vi "Log Data.vi"(8 "error in (no error)":errorcluster, 9 "variant":variant, 10 "Data REF":T1, 11 "Logging Configuration":T2={"Log File Base Path"=path "", "TDMS File Reference"=refnum, "Reset"=FALSE, "Wait"=0.0, "Start Time"=0.0, "Update Rate"=1, "Channel Names"=[], "System Preset"=variant} {"Update Rate" min=1 max=10 step=1}) -> (0 "error out":errorcluster)   [LabVIEW 2020, in "SAVE.lvlib"]
doc: "This VI uses the TDMS Write function to write data to a TDMS file."
uses:
  SAVE.lvlib
  Save Configuration.ctl
  support/PCT Data REFs.ctl
  <instrlib>/PalmSens SDK for LabVIEW 5.10/PalmSens/MeasurementResults.ctl
  <instrlib>/PalmSens SDK for LabVIEW 5.10/PalmSens/LiveCurveResult.ctl
  support/PCT FGV CMD.ctl
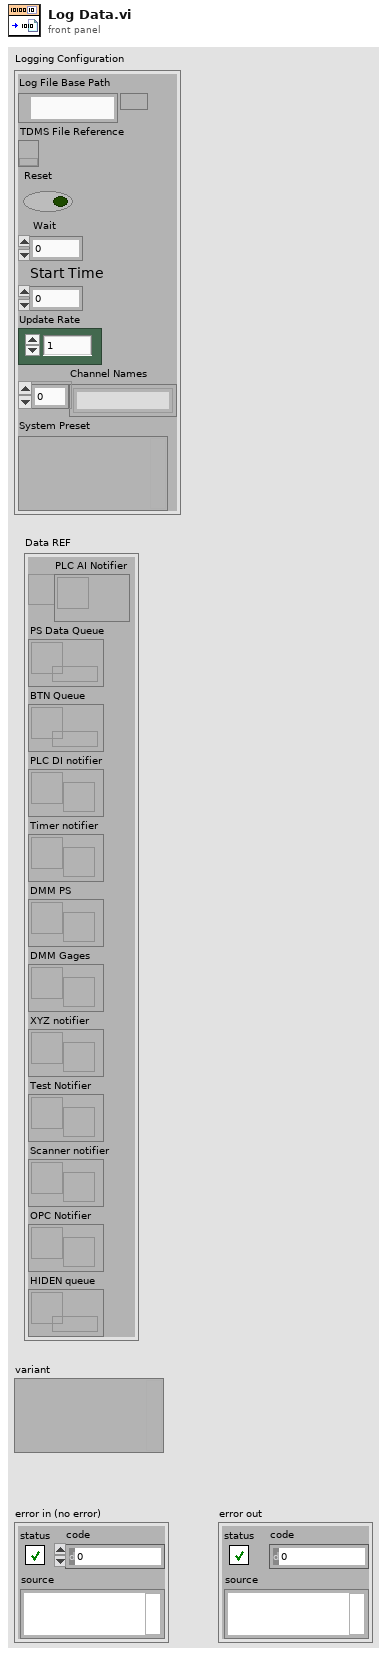
[diagram p1: front panel]
types:
  T1 = typedef "PCT Data REFs.ctl" = cluster{"PLC AI Notifier":refnum<notifier>, "PS Data Queue":refnum<queue>, "BTN Queue":refnum<queue>, "PLC DI notifier":refnum<notifier>, "Timer notifier":refnum<notifier>, "DMM PS":refnum<notifier>, "DMM Gages":refnum<notifier>, "XYZ notifier":refnum<notifier>, "Test Notifier":refnum<notifier>, "Scanner notifier":refnum<notifier>, "OPC Notifier":refnum<notifier>, "HIDEN queue":refnum<queue>}
  T2 = typedef "SAVE.lvlib/Save Configuration.ctl" = cluster{"Log File Base Path":path, "TDMS File Reference":refnum<k34>, "Reset":bool, "Wait":dbl, "Start Time":dbl, "Update Rate":u16, "Channel Names":string[], "System Preset":variant}
  T3 = typedef "MeasurementResults.ctl" = T4[]
  T4 = typedef "LiveCurveResult.ctl" = cluster{"X Label":string, "Y Label":string, "Name":string, "Index":i16, "Curve Values":cluster{"Values":cluster{"X Value":dbl, "Y Value":dbl}[], "Index":i16}}
  T5 = cluster{"whole match":string, "Results":T3, "Measurements":dbl[]}
  T6 = typedef "PCT FGV CMD.ctl" = enum16{"INIT", "GET", "SET"}
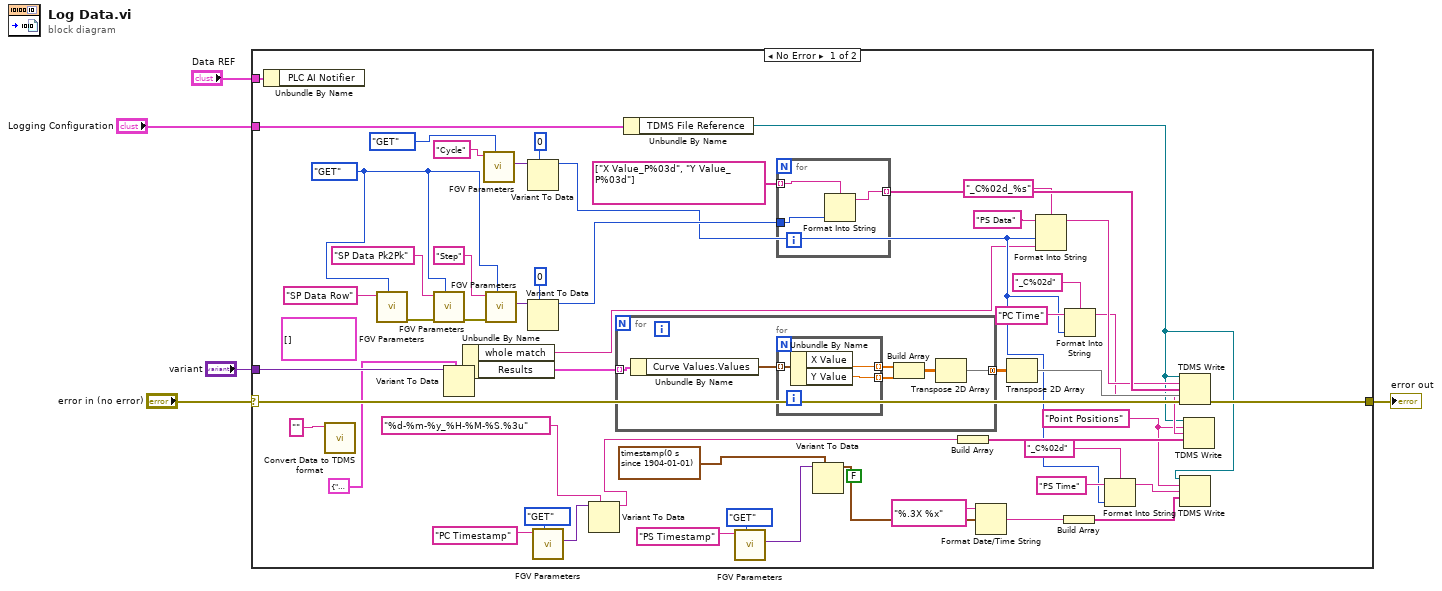
[diagram p0: block diagram]
diagram:
  n1 = case shown="No Error" "error in (no error)" {
    selector: "error in (no error)" -> [w56 w71]
    tunnel: "Logging Configuration" -> [w58 _]
    tunnel: [w40 w71] -> w4
    tunnel: "Data REF" -> [w57 _]
    tunnel: "variant" -> [w54 _]
    frame No Error {
      (unwired) FALSE ("want seconds? (F)")
      w21 = "Point Positions" ("channel name(s) in (Untitled)")
      (unwired) T3 [] ("Results")
      w49 = PCT_FGV_CMD."GET" ("CMD")
      n2 = Unbundle By Name(w57) -> ()  [unwired: 1 out]
      n3 = call "Convert Data to TDMS format.vi"("Mode"="") -> ()  [unwired: 9 in, 2 out]
      n4 = call "FGV Parameters.vi"("CMD"=w49, "Key"="SP Data Row") -> ("error out"=w53:errorcluster)  [unwired: 7 in, 2 out]
      n5 = call "FGV Parameters.vi"("CMD"=w49, "error in (no error)"=w53, "Key"="SP Data Pk2Pk") -> ("error out"=w50:errorcluster)  [unwired: 6 in, 2 out]
      n6 = Variant To Data(type=T5 {"whole match"="", "Results"=[], "Measurements"=[]} ("output cluster"), Variant=w54) -> (data=w39:T5)  [unwired: 1 in, 1 out]
      n7 = Unbundle By Name(w39) -> ("whole match"=w6:string, "Results"=w7:T3)
      n8 = call "FGV Parameters.vi"("CMD"=PCT_FGV_CMD."GET", "Key"="Cycle") -> ("output"=w41:variant)  [unwired: 7 in, 2 out]
      n9 = call "FGV Parameters.vi"("CMD"=w49, "error in (no error)"=w50, "Key"="Step") -> ("output"=w46:variant)  [unwired: 6 in, 2 out]
      n10 = Variant To Data(type=0 ("current Step"), Variant=w41) -> (data=w17:i32)  [unwired: 1 in, 1 out]
      n11 = Variant To Data(type=0 ("current Step"), Variant=w46) -> (data=w35:i32)  [unwired: 1 in, 1 out]
      n12 = call "FGV Parameters.vi"("CMD"=PCT_FGV_CMD."GET", "Key"="PC Timestamp") -> ("output"=w11:variant)  [unwired: 7 in, 2 out]
      n13 = Variant To Data(type="%d-%m-%y_%H-%M-%S.%3u" ("time format string (%c)"), Variant=w11) -> (data=w9:string)  [unwired: 1 in, 1 out]
      n14 = for {
        tunnel: w7 -> [w67] mode=indexing
        tunnel: [w62] -> w48 mode=concatenating
        n15 = Unbundle By Name(w67) -> ("Curve Values.Values"=w65:cluster{"X Value":dbl, "Y Value":dbl}[])
        n16 = for {
          tunnel: [w70] -> w66 mode=indexing
          tunnel: w65 -> [w69] mode=indexing
          tunnel: [w68] -> w63 mode=indexing
          n17 = Unbundle By Name(w69) -> ("X Value"=w70:dbl, "Y Value"=w68:dbl)
        }
        n18 = Build Array(w66, w63) -> (w64:dbl[][])
        n19 = Transpose 2D Array(2D array=w64) -> (transposed array=w62:dbl[][])
      }
      n20 = Unbundle By Name(w58) -> ("TDMS File Reference"=w20:refnum<k34>)
      n21 = call "FGV Parameters.vi"("CMD"=PCT_FGV_CMD."GET", "Key"="PS Timestamp") -> ("output"=w25:variant)  [unwired: 7 in, 2 out]
      n22 = for {
        tunnel: string[] ["X Value_P%03d", "Y Value_P%03d"] ("format string") -> [w61] mode=indexing
        tunnel: w35 -> [w60]
        tunnel: [w59] -> w34 mode=indexing
        n23 = Format Into String(format string=w61, w60) -> (resulting string=w59:string)  [unwired: 2 in, 1 out]
      }
      n24 = Variant To Data(type=timestamp(0 s since 1904-01-01) ("TimeStamp 2"), Variant=w25) -> (data=w22:timestamp)  [unwired: 1 in, 1 out]
      n25 = Build Array(w9) -> (w38:string[])
      n26 = Format Date/Time String(time format string (%c)="%.3X %x", seconds (now)=w22) -> (date/time string=w15:string)  [unwired: 1 in]
      n27 = Transpose 2D Array(2D array=w48) -> (transposed array=w37:dbl[][])
      n28 = Format Into String(format string="_C%02d_%s", initial string="PS Data" ("group name in (Untitled)"), w17, w6) -> (resulting string=w32:string)  [unwired: 1 in, 1 out]
      n29 = Build Array(w15) -> (w14:string[])
      n30 = Format Into String(format string="_C%02d", initial string="PC Time" ("channel name(s) in (Untitled)"), w17) -> (resulting string=w28:string)  [unwired: 1 in, 1 out]
      n31 = Format Into String(format string="_C%02d", initial string="PS Time" ("channel name(s) in (Untitled)"), w17) -> (resulting string=w16:string)  [unwired: 1 in, 1 out]
      n32 = TDMS Write(0:w20, 5:w32, 7:w34, 9:w37, 11:w56) -> (15:w40:errorcluster)  [unwired: 1 in, 3 out]
      n33 = TDMS Write(0:w20, 5:w21, 7:w16, 9:w14) -> ()  [unwired: 2 in, 4 out]
      n34 = TDMS Write(0:w20, 5:w21, 7:w28, 9:w38) -> ()  [unwired: 2 in, 4 out]
    }
    frame Error {
    }
  }
  "error out" <- w4
